vi "DiffDriveCtrl_example.vi"() -> ()   [LabVIEW 2019]
uses:
  <vilib>/Rock Robotics/WPI/ThirdParty/JAS_Junk/TrajLib/TypeDef/DIFF_DRIVE_TRAIN_SIM.ctl
  <vilib>/Rock Robotics/WPI/ThirdParty/JAS_Junk/TrajLib/TypeDef/LINEAR_SYSTEM.ctl
  <vilib>/Analysis/Matrix/Datatypes/RealMatrix.ctl
  <vilib>/Rock Robotics/WPI/ThirdParty/JAS_Junk/TrajLib/TypeDef/DCMOTOR.CTL
  <vilib>/Rock Robotics/WPI/ThirdParty/JAS_Junk/TrajLib/Enum/DCMOTOR_TYPES_ENUM.ctl
  <vilib>/Rock Robotics/WPI/ThirdParty/JAS_Junk/TrajLib/Enum/DIFF_DRIVE_TRAIN_SIM_STATE_ENUM.ctl
  <vilib>/Rock Robotics/WPI/ThirdParty/JAS_Junk/TrajLib/Enum/DIFF_DRIVE_ToughBoxMini_GearChoice_ENUM.ctl
  <vilib>/Rock Robotics/WPI/ThirdParty/JAS_Junk/TrajLib/Enum/DIFF_DRIVE_KitBot_WheelSize_ENUM.ctl
  <vilib>/Rock Robotics/WPI/ThirdParty/JAS_Junk/TrajLib/VI/numCmd_ObtainQueue_TwoDbl.vi
  <vilib>/Rock Robotics/WPI/ThirdParty/JAS_Junk/TrajLib/LinearSystemId_CreateDriveTrainVelocitySystem.vi
  <vilib>/Rock Robotics/WPI/ThirdParty/JAS_Junk/TrajLib/DCMotor_PickMotor.vi
  <vilib>/Rock Robotics/WPI/ThirdParty/JAS_Junk/TrajLib/BatterySim_CalculateLoadedBatteryVoltage.vi
  <vilib>/Rock Robotics/WPI/ThirdParty/JAS_Junk/TrajLib/LinearSystem_New.vi
  <vilib>/Rock Robotics/WPI/ThirdParty/JAS_Junk/TrajLib/MatBuilder_Create.vi
  <vilib>/Rock Robotics/WPI/ThirdParty/JAS_Junk/TrajLib/MatBuilder_Fill.vi
  <vilib>/Rock Robotics/WPI/ThirdParty/JAS_Junk/TrajLib/MatrixHelper_Zero.vi
  <vilib>/Rock Robotics/WPI/ThirdParty/JAS_Junk/TrajLib/DCMotor_GetCIM.vi
  <vilib>/Rock Robotics/WPI/ThirdParty/JAS_Junk/TrajLib/DCMotor_GetAndymark9015.vi
  <vilib>/Rock Robotics/WPI/ThirdParty/JAS_Junk/TrajLib/DCMotor_GetAndymarkRs775_125.vi
  <vilib>/Rock Robotics/WPI/ThirdParty/JAS_Junk/TrajLib/DCMotor_GetBag.vi
  <vilib>/Rock Robotics/WPI/ThirdParty/JAS_Junk/TrajLib/DCMotor_GetBanebotsRs550.vi
  <vilib>/Rock Robotics/WPI/ThirdParty/JAS_Junk/TrajLib/DCMotor_GetBanebotsRs775.vi
  <vilib>/Rock Robotics/WPI/ThirdParty/JAS_Junk/TrajLib/DCMotor_GetFalcon500.vi
  <vilib>/Rock Robotics/WPI/ThirdParty/JAS_Junk/TrajLib/DCMotor_GetMiniCIM.vi
  <vilib>/Rock Robotics/WPI/ThirdParty/JAS_Junk/TrajLib/DCMotor_GetNEO.vi
  <vilib>/Rock Robotics/WPI/ThirdParty/JAS_Junk/TrajLib/DCMotor_GetNEO550.vi
  <vilib>/Rock Robotics/WPI/ThirdParty/JAS_Junk/TrajLib/DCMotor_GetRomiBuiltIn.vi
  <vilib>/Rock Robotics/WPI/ThirdParty/JAS_Junk/TrajLib/DCMotor_GetVex775Pro.vi
  <vilib>/Rock Robotics/WPI/ThirdParty/JAS_Junk/TrajLib/VI/DCMotor_GetAndymarkAM2235A.vi
  <vilib>/Rock Robotics/WPI/ThirdParty/JAS_Junk/TrajLib/VI/DCMotor_GetAndymarkAM3493.vi
  <vilib>/Rock Robotics/WPI/ThirdParty/JAS_Junk/TrajLib/MatrixHelper_CoerceSize.vi
  <vilib>/Rock Robotics/WPI/ThirdParty/JAS_Junk/TrajLib/DCMotor_New.vi
  <vilib>/Rock Robotics/WPI/ThirdParty/JAS_Junk/TrajLib/VI/Units_RotationsPerMinuteToRadiansPerSecond.vi
  <vilib>/Rock Robotics/WPI/ThirdParty/JAS_Junk/TrajLib/Trajectory_Library.lvlib
  <vilib>/Analysis/Matrix/NI_Matrix.lvlib
panel:
  in  "Tab Control":enum32{"Control", "Simulation"}(tab)
  out "Right Motor Dmd":dbl format="%20.3f"
  out "Left Motor Dmd":dbl format="%20.3f"
  in  "Speed Demand\nFt/Sec":dbl(slide) scale=-10.0..10.0
  out "Left Motor Vel - PV (Ft/Sec)":dbl format="%20.3f"
  out "Right Motor Vel - PV (Ft/Sec)":dbl format="%20.3f"
  out "Battery Voltage (Volts)":dbl format="%20.3f"
  out "Voltage, Current Chart":cluster{dbl, dbl, "Voltage":dbl}(graph)
  out "PV, SP Chart":T1(graph)
  out "Motor Current  - Left (Amps)":dbl format="%20.3f"
  out "Motor Current  - Right (Amps)":dbl format="%20.3f"
  out "Right Motor Dist (Ft)":dbl format="%20.3f"
  out "Left Motor Dist (Ft)":dbl format="%20.3f"
  out "Gyro Heading (Deg)":dbl format="%20.3f"
  out "Differential Drive Train Sim":T2 {"m_Motor"."Jr_KgM2" format="%13.5p"; "m_Motor"."L_H" format="%13.5p"; "m_Motor"."Kt_NMPerAmp" format="%13.5p"; "m_Motor"."KvINV_RadPerSecPerVolt" format="%13.5p"; "m_Motor"."R_Ohms" format="%13.5p"; "m_Motor"."FreeSpeed_RadPerSec" format="%13.5p"; "m_Motor"."FreeCurrent_Amps" format="%13.5p"; "m_Motor"."StallCurrent_Amps" format="%13.5p"; "m_Motor"."StallTorque_NM" format="%13.5p"; "m_Motor"."nominalVoltage_Volts" format="%13.5p"}
  # "<States, 1>"
  # "<Outputs, 1>"
  # "<Inputs, 1>"
  # "<Outputs, 1>"
  # "<States,States>"
  # "<States,Inputs>"
  # "<Outputs,States>"
  # "<Outputs,Inputs>"
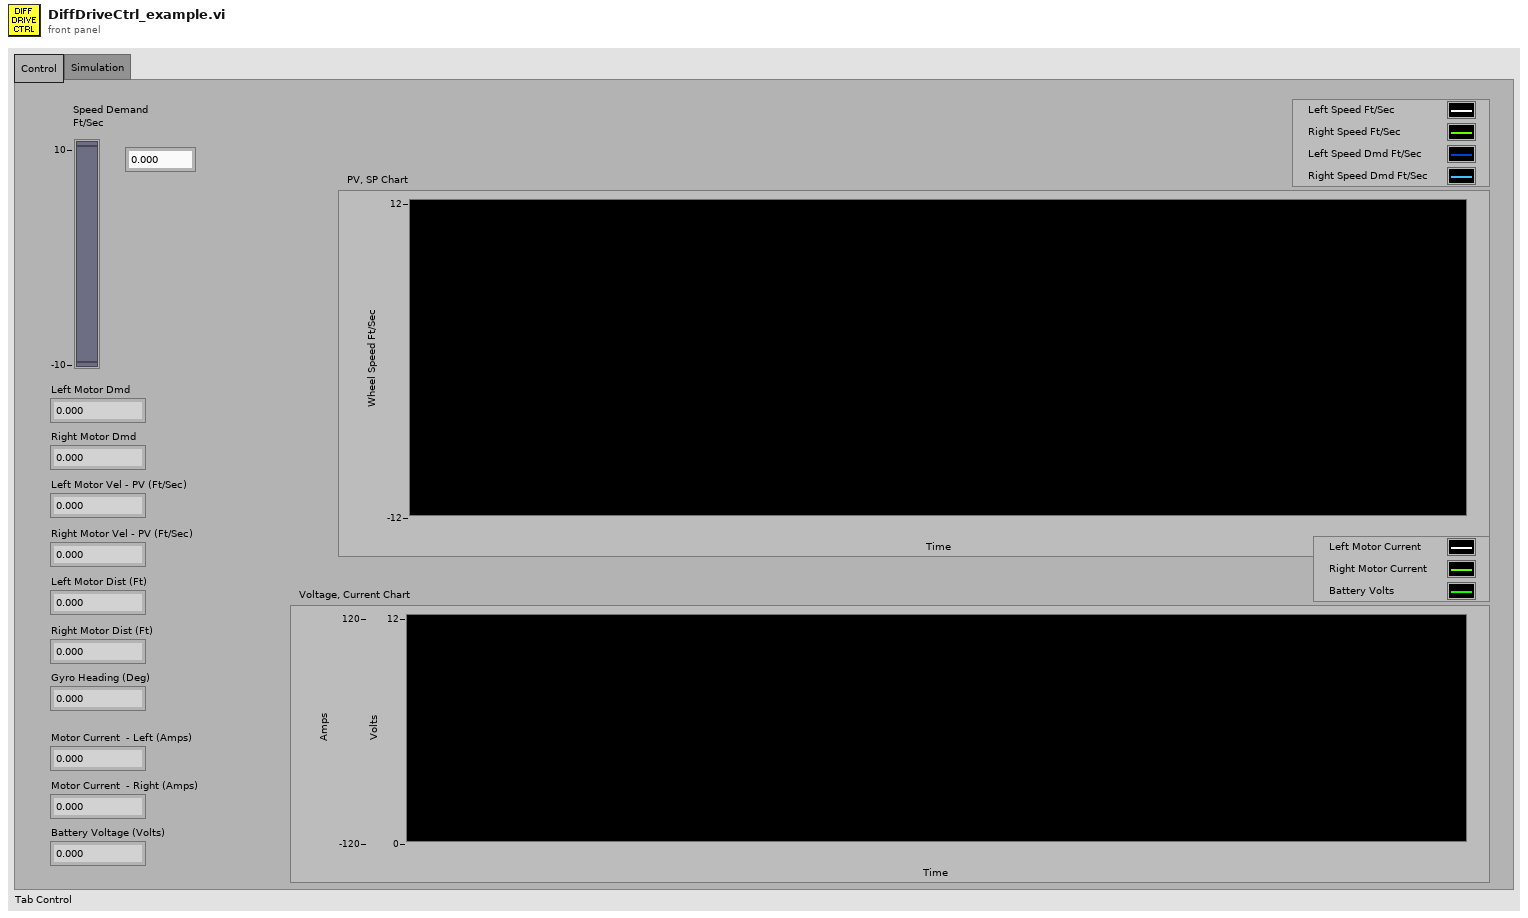
[diagram p1: front panel]
types:
  T1 = cluster{"Feet":dbl, "Feet":dbl, "Value 1":dbl, "Value 2":dbl}
  T2 = typedef "Trajectory_Library.lvlib/DIFF_DRIVE_TRAIN_SIM.ctl" = cluster{"m_Plant":T3, "m_X":T4, "m_Y":T4, "m_U":T4, "MeasureStdDev":T4, "m_Motor":T5, "m_OriginalGearing":dbl, "m_CurrentGearing":dbl, "m_WheelRadius_M":dbl, "m_RB":dbl}
  T3 = typedef "Trajectory_Library.lvlib/LINEAR_SYSTEM.ctl" = cluster{"m_A":T4, "m_B":T4, "m_C":T4, "m_D":T4, "States":i32, "Inputs":i32, "Outputs":i32}
  T4 = typedef "NI_Matrix.lvlib/RealMatrix.ctl" = dbl[][]
  T5 = typedef "Trajectory_Library.lvlib/DCMOTOR.CTL" = cluster{"nominalVoltage_Volts":dbl, "StallTorque_NM":dbl, "StallCurrent_Amps":dbl, "FreeCurrent_Amps":dbl, "FreeSpeed_RadPerSec":dbl, "R_Ohms":dbl, "KvINV_RadPerSecPerVolt":dbl, "Kt_NMPerAmp":dbl, "L_H":dbl, "Jr_KgM2":dbl}
  T6 = typedef "Trajectory_Library.lvlib/DIFF_DRIVE_TRAIN_SIM_STATE_ENUM.ctl" = enum16{"X_POS", "Y_POS", "HEADING", "LEFT_VEL", "RIGHT_VEL", "LEFT_DIST", "RIGHT_DIST"}
  T7 = typedef "Trajectory_Library.lvlib/DIFF_DRIVE_KitBot_WheelSize_ENUM.ctl" = enum16{"4 Inch", "6 Inch", "8 Inch", "10 Inch"}
  T8 = typedef "Trajectory_Library.lvlib/DIFF_DRIVE_ToughBoxMini_GearChoice_ENUM.ctl" = enum16{"Ratio_12_75", "Ratio_10_71", "Ratio_8_45", "Ratio_7_31", "Ratio_5_95"}
  T9 = typedef "Trajectory_Library.lvlib/DCMOTOR_TYPES_ENUM.ctl" = enum16{"CIM", "AndyMark 9015", "Andy Mark RS 775 125", "Bag", "BaneBots RS 550", "BaneBots RS 775", "Falcon 500", "Mini CIM", "NEO", "NEO 550", "Romi BuiltIn", "Vex 775 Pro", "Snow Blower AM 2235A", "Bosch Seat AM 3493"}
  T10 = typedef "Trajectory_Library.lvlib/DIFF_DRIVE_SIM_SIMULATION_PARAMS.ctl" = cluster{"X Pos Meas Std Dev M":dbl, "Y Pos Meas Std Dev M":dbl, "Heading Meas Std Dev Rad":dbl, "Left Vel Meas Std Dev M/S":dbl, "Right Vel Meas Std Dev M/S":dbl, "Left Pos Meas Std Dev M":dbl, "Right Pos Meas Std Dev M":dbl}
  T11 = typedef "Trajectory_Library.lvlib/DIFF_DRIVE_SIM_MODEL_PARAMS.CTL" = cluster{"TracWidth_M":dbl, "WheelRadius_M":dbl, "Gearing":dbl, "Mass kg":dbl, "MOI kgm2":dbl, "DCMOTOR_TYPES":T9, "Num Motors":i32}
  T12 = typedef "Trajectory_Library.lvlib/LINEAR_SYSTEM_LOOP_DIFF_DRV_CTRL_PARAMS.CTL" = cluster{"Left Vel Model Std Dev m/s":dbl, "Left Vel Meas Std Dev m/s":dbl, "Left Vel Ctrl Tol m/s":dbl, "Max Control Effort":dbl, "Right Vel Ctrl Tol m/s":dbl, "Right Vel Meas Std Dev m/s":dbl, "Right Vel Model Std Dev m/s":dbl}
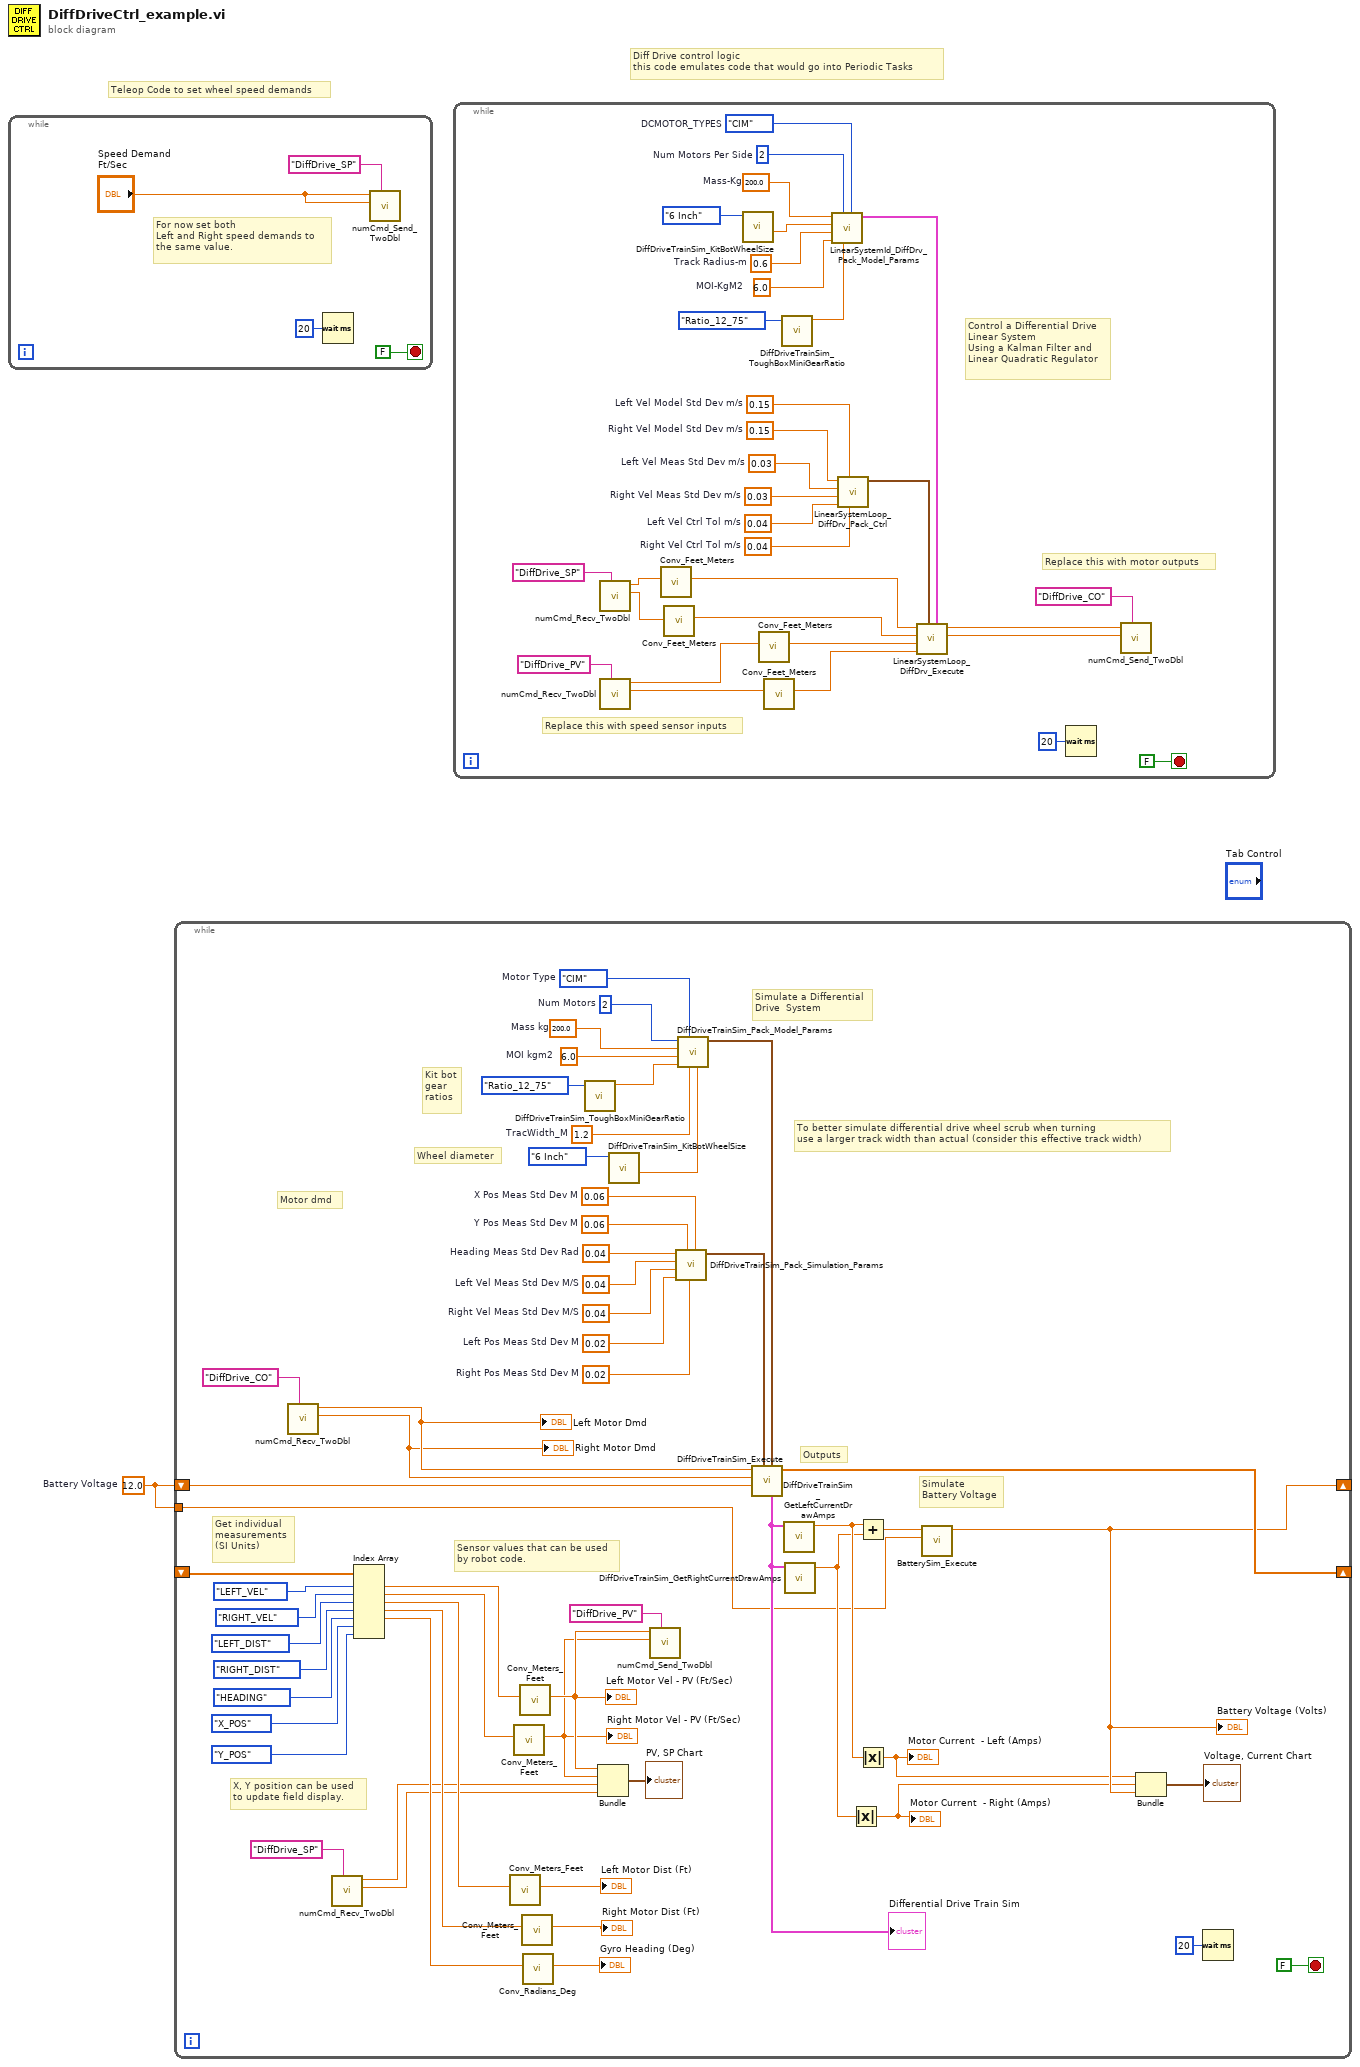
[diagram p0: block diagram]
diagram:
  w1 = 12.0  # Battery Voltage
  # "Teleop Code to set wheel speed demands"
  # "Diff Drive control logic\nthis code emulates code that would go into Periodic Tasks"
  n1 = while {
    stop <- FALSE stop-if-true
    # "For now set both\nLeft and Right speed demands to\nthe same value."
    n2 = Wait (ms)(milliseconds to wait=u32 20) -> ()  [unwired: 1 out]
    n3 = call <vilib>:"numCmd_Send_TwoDbl.vi"("Command Name"="DiffDrive_SP", "Value 2"="Speed Demand\nFt/Sec", "Value 1"="Speed Demand\nFt/Sec") -> ()  [unwired: 8 in, 1 out]
  }
  n4 = while {
    shift-right: [w33] -> _
    shift-left: w1 -> [w34]
    shift-right: [w58] -> _
    shift-left: _ -> [w42]
    tunnel: w1 -> [w17]
    stop <- FALSE stop-if-true
    w46 = 200.0  # Mass kg
    w47 = 6.0  # MOI kgm2
    w48 = 1.2  # TracWidth_M
    w49 = 0.04  # Heading Meas Std Dev Rad
    w50 = 0.04  # Left Vel Meas Std Dev M/S
    w51 = 0.04  # Right Vel Meas Std Dev M/S
    w52 = 0.02  # Left Pos Meas Std Dev M
    w53 = 0.06  # Y Pos Meas Std Dev M
    w54 = 0.02  # Right Pos Meas Std Dev M
    w55 = 0.06  # X Pos Meas Std Dev M
    w61 = 2  # Num Motors
    w62 = DCMOTOR_TYPES_ENUM."CIM"  # Motor Type
    # "To better simulate differential drive wheel scrub when turning\nuse a larger track width than actual (consider this effective track width)"
    # "Sensor values that can be used\nby robot code."
    # "X, Y position can be used\nto update field display."
    # "Motor dmd"
    # "Wheel diameter"
    # "Get individual\nmeasurements\n(SI Units)"
    # "Kit bot\ngear \nratios"
    # "Outputs"
    # "Simulate\nBattery Voltage"
    # "Simulate a Differential\nDrive  System"
    n5 = call <vilib>:"numCmd_Recv_TwoDbl.vi"("Command Name"="DiffDrive_CO") -> ("Value 2"=w6:dbl, "Value 1"=w7:dbl)  [unwired: 7 in, 2 out]
    "Left Motor Dmd" <- w7
    "Right Motor Dmd" <- w6
    n6 = call <vilib>:"numCmd_Recv_TwoDbl.vi"("Command Name"="DiffDrive_SP") -> ("Value 2"=w11:dbl, "Value 1"=w12:dbl)  [unwired: 7 in, 2 out]
    n7 = Index Array(array=w42, index #1=DIFF_DRIVE_TRAIN_SIM_STATE_ENUM."LEFT_VEL" ("DIFF_DRIVE_TRAIN_SIM_STATE"), index #2=DIFF_DRIVE_TRAIN_SIM_STATE_ENUM."RIGHT_VEL" ("DIFF_DRIVE_TRAIN_SIM_STATE"), index #3=DIFF_DRIVE_TRAIN_SIM_STATE_ENUM."LEFT_DIST" ("DIFF_DRIVE_TRAIN_SIM_STATE"), index #4=DIFF_DRIVE_TRAIN_SIM_STATE_ENUM."RIGHT_DIST" ("DIFF_DRIVE_TRAIN_SIM_STATE"), index #5=DIFF_DRIVE_TRAIN_SIM_STATE_ENUM."HEADING" ("DIFF_DRIVE_TRAIN_SIM_STATE"), index #6=DIFF_DRIVE_TRAIN_SIM_STATE_ENUM."X_POS" ("DIFF_DRIVE_TRAIN_SIM_STATE"), index #7=DIFF_DRIVE_TRAIN_SIM_STATE_ENUM."Y_POS" ("DIFF_DRIVE_TRAIN_SIM_STATE")) -> (element #1=w31:dbl, element #2=w30:dbl, element #3=w27:dbl, element #4=w26:dbl, element #5=w18:dbl)  [unwired: 2 out]
    n8 = call <vilib>:"Conv_Meters_Feet.vi"("Meters"=w27) -> ("Feet"=→"Left Motor Dist (Ft)":dbl)  [unwired: 10 in]
    n9 = call <vilib>:"Conv_Meters_Feet.vi"("Meters"=w30) -> ("Feet"=w8:dbl)  [unwired: 10 in]
    "Right Motor Vel - PV (Ft/Sec)" <- w8
    n10 = call <vilib>:"Conv_Meters_Feet.vi"("Meters"=w31) -> ("Feet"=w9:dbl)  [unwired: 10 in]
    "Left Motor Vel - PV (Ft/Sec)" <- w9
    n11 = call <vilib>:"Conv_Meters_Feet.vi"("Meters"=w26) -> ("Feet"=→"Right Motor Dist (Ft)":dbl)  [unwired: 10 in]
    n12 = call <vilib>:"Conv_Radians_Deg.vi"("Radians"=w18) -> ("Degrees"=→"Gyro Heading (Deg)":dbl)  [unwired: 10 in]
    n13 = call <vilib>:"DiffDriveTrainSim_ToughBoxMiniGearRatio.vi"("ToughBoxMiniGear"=DIFF_DRIVE_ToughBoxMini_GearChoice_ENUM."Ratio_12_75") -> ("GearRatio"=w44:dbl)  [unwired: 10 in]
    n14 = Bundle("Feet"=w9, "Feet"=w8, "Value 1"=w12, "Value 2"=w11) -> (→"PV, SP Chart":T1)  [unwired: 1 in]
    n15 = call <vilib>:"DiffDriveTrainSim_KitBotWheelSize.vi"("Wheel Size"=DIFF_DRIVE_KitBot_WheelSize_ENUM."6 Inch") -> ("WheelRadius_M"=w35:dbl)  [unwired: 9 in, 1 out]
    n16 = call <vilib>:"numCmd_Send_TwoDbl.vi"("Command Name"="DiffDrive_PV", "Value 2"=w8, "Value 1"=w9) -> ()  [unwired: 8 in, 1 out]
    n17 = call <vilib>:"DiffDriveTrainSim_Pack_Simulation_Params.vi"("X Pos Meas Std Dev M"=w55, "Right Pos Meas Std Dev M"=w54, "Y Pos Meas Std Dev M"=w53, "Left Pos Meas Std Dev M"=w52, "Right Vel Meas Std Dev M/S"=w51, "Left Vel Meas Std Dev M/S"=w50, "Heading Meas Std Dev Rad"=w49) -> ("DiffDriveSim_Simulation _Params"=w56:T10)  [unwired: 4 in]
    n18 = call <vilib>:"DiffDriveTrainSim_Pack_Model_Params.vi"("WheelRadius_M"=w35, "TracWidth_M"=w48, "DCMOTOR_TYPES"=w62, "Gearing"=w44, "MOI kgm2"=w47, "Mass kg"=w46, "Num Motors"=w61) -> ("DiffDriveSim_Model _Params"=w57:T11)  [unwired: 4 in]
    n19 = call <vilib>:"DiffDriveTrainSim_Execute.vi"("LinearSystem_ID_DiffDrv_Model"=w57, "DiffDriveSim_Simulation _Params"=w56, "BatteryVoltage"=w34, "Right Motor Dmd"=w6, "Left Motor Dmd"=w7) -> ("Outputs"=w58:dbl[], "out DiffDriveTrainSim"=w32:T2)  [unwired: 4 in, 1 out]
    "Differential Drive Train Sim" <- w32
    n20 = call <vilib>:"DiffDriveTrainSim_GetLeftCurrentDrawAmps.vi"("DiffDriveTrainSim"=w32) -> ("LeftCurrentDraw_Amps"=w22:dbl)  [unwired: 10 in]
    n21 = call <vilib>:"DiffDriveTrainSim_GetRightCurrentDrawAmps.vi"("DiffDriveTrainSim"=w32) -> ("RightCurrentDraw_Amps"=w21:dbl)  [unwired: 10 in]
    n22 = Absolute Value(x=w21) -> (abs(x)=w19:dbl)
    "Motor Current  - Right (Amps)" <- w19
    n23 = Add(x=w22, y=w21) -> (x+y=w43:dbl)
    n24 = Absolute Value(x=w22) -> (abs(x)=w20:dbl)
    "Motor Current  - Left (Amps)" <- w20
    n25 = call <vilib>:"BatterySim_Execute.vi"("Nominal Battery Voltage"=w17, "Current"=w43) -> ("Voltage"=w33:dbl)  [unwired: 9 in]
    "Battery Voltage (Volts)" <- w33
    n26 = Bundle(w20, w19, "Voltage"=w33) -> (→"Voltage, Current Chart":cluster{dbl, dbl, "Voltage":dbl})  [unwired: 1 in]
    n27 = Wait (ms)(milliseconds to wait=u32 20) -> ()  [unwired: 1 out]
  }
  n28 = while {
    stop <- FALSE stop-if-true
    w80 = 0.15  # Right Vel Model Std Dev m/s
    w81 = 0.03  # Left Vel Meas Std Dev m/s
    w82 = 0.03  # Right Vel Meas Std Dev m/s
    w83 = 0.04  # Left Vel Ctrl Tol m/s
    w84 = 0.15  # Left Vel Model Std Dev m/s
    w85 = 0.04  # Right Vel Ctrl Tol m/s
    w86 = 200.0  # Mass-Kg
    w87 = 0.6  # Track Radius-m
    w88 = 6.0  # MOI-KgM2
    w89 = 2  # Num Motors Per Side
    w90 = DCMOTOR_TYPES_ENUM."CIM"  # DCMOTOR_TYPES
    # "Replace this with speed sensor inputs"
    # "Replace this with motor outputs"
    # "Control a Differential Drive\nLinear System\nUsing a Kalman Filter and \nLinear Quadratic Regulator"
    n29 = call <vilib>:"numCmd_Recv_TwoDbl.vi"("Command Name"="DiffDrive_SP") -> ("Value 2"=w75:dbl, "Value 1"=w76:dbl)  [unwired: 7 in, 2 out]
    n30 = call <vilib>:"numCmd_Recv_TwoDbl.vi"("Command Name"="DiffDrive_PV") -> ("Value 2"=w70:dbl, "Value 1"=w71:dbl)  [unwired: 7 in, 2 out]
    n31 = call <vilib>:"Conv_Feet_Meters.vi"("Feet"=w76) -> ("Meters"=w79:dbl)  [unwired: 10 in]
    n32 = call <vilib>:"Conv_Feet_Meters.vi"("Feet"=w75) -> ("Meters"=w78:dbl)  [unwired: 10 in]
    n33 = call <vilib>:"DiffDriveTrainSim_KitBotWheelSize.vi"("Wheel Size"=DIFF_DRIVE_KitBot_WheelSize_ENUM."6 Inch") -> ("WheelRadius_M"=w63:dbl)  [unwired: 9 in, 1 out]
    n34 = call <vilib>:"Conv_Feet_Meters.vi"("Feet"=w71) -> ("Meters"=w74:dbl)  [unwired: 10 in]
    n35 = call <vilib>:"Conv_Feet_Meters.vi"("Feet"=w70) -> ("Meters"=w73:dbl)  [unwired: 10 in]
    n36 = call <vilib>:"DiffDriveTrainSim_ToughBoxMiniGearRatio.vi"("ToughBoxMiniGear"=DIFF_DRIVE_ToughBoxMini_GearChoice_ENUM."Ratio_12_75") -> ("GearRatio"=w65:dbl)  [unwired: 10 in]
    n37 = call <vilib>:"LinearSystemId_DiffDrv_Pack_Model_Params.vi"("DCMOTOR_TYPES"=w90, "Gear Ratio"=w65, "Num Motors Per Side"=w89, "MOI-KgM2"=w88, "Track Radius-m"=w87, "Wheel Radius-M"=w63, "Mass-Kg"=w86) -> ("DiffDrv_LinearSystem"=w91:T3)  [unwired: 4 in]
    n38 = call <vilib>:"LinearSystemLoop_DiffDrv_Pack_Ctrl.vi"("Right Vel Ctrl Tol m/s"=w85, "Left Vel Model Std Dev m/s"=w84, "Left Vel Ctrl Tol m/s"=w83, "Right Vel Meas Std Dev m/s"=w82, "Left Vel Meas Std Dev m/s"=w81, "Right Vel Model Std Dev m/s"=w80) -> ("LinearSystemLoop_DiffDrv_Ctrl_Params"=w92:T12)  [unwired: 5 in]
    n39 = call <vilib>:"LinearSystemLoop_DiffDrv_Execute.vi"("Linear System"=w91, "LinearSystemLoop_DiffDrv_Control_Params"=w92, "Right Vel PV m/s"=w73, "Left Vel PV m/s"=w74, "Right Vel SP m/s"=w78, "Left Vel SP m/s"=w79) -> ("Right Motor Dmd"=w67:dbl, "Left Motor Dmd"=w68:dbl)  [unwired: 1 in, 3 out]
    n40 = Wait (ms)(milliseconds to wait=u32 20) -> ()  [unwired: 1 out]
    n41 = call <vilib>:"numCmd_Send_TwoDbl.vi"("Command Name"="DiffDrive_CO", "Value 2"=w67, "Value 1"=w68) -> ()  [unwired: 8 in, 1 out]
  }
